vi "spectrum_display.vi"(4 "Chart data?":bool, 5 "Modulation info":T8 {"Hi channels at low" min=0 step=1; "Low carriers" format="%#_6p"; "High carriers" format="%#_6p"}, 6 "Reset STFT":bool, 7 "Config":T2={"IO params"={"Conversion"={"Rate"=0.0, "Num cards"=0, "Out channels"=4}, "Carriers"={"Phase shift"=180.0, "Levels"=[[0.8, 0.8, 0.8], [0.03, 0.03, 0.03]], "Delay samples"=73.15}, "TCP"={"Host"="192.168.1.15", "Port"=6666, "Buffering"=6, "Timeout"=6}, "Input channel sign"=[1, 1, 1]}, "High rate STFT"={"Win param"=0.0, "Window type"=0, "Win order"=0, "DFT size"=0, "Channels"=[], "Oversample"=0}, "Low rate STFT"={"Win param"=0.0, "Window type"=0, "Win order"=0, "DFT size"=0, "Channels"=[], "Oversample"=0}, "Filtering "=[]} {"Filtering"."Distortion"."Limit" format="%#_3p"; "Filtering"."Distortion"."LF cut" format="%#_3p"; "Filtering"."Kalman"."Measure noise" format="%#_3p"; "Filtering"."Kalman"."Process noise" format="%#_3p"; "Filtering"."Hum"."Limit" format="%#_3p"; "Filtering"."Hum"."Frequency" format="%#_4p"; "Low rate STFT"."Oversample" min=1 step=1; "Low rate STFT"."Channels" min=0 step=1; "Low rate STFT"."DFT size" min=1 step=1; "Low rate STFT"."Window type" items=["Rectangle"=0, "Hanning"=1, "Hamming"=2, "Blackman-Harris"=3, "Exact Blackman"=4, "Blackman"=5, "Flat Top"=6, "4 Term B-Harris "=7, "7 Term B-Harris"=8, "Low Sidelobe"=9, "Blackman Nuttall"=11, "Triangle"=30, "Bartlett-Hanning"=31, "Bohman"=32, "Parzen"=33, "Welch"=34, "Kaiser"=60, "Dolph-Chebyshev"=61, "Gaussian"=62]; "High rate STFT"."Oversample" min=1 step=1; "High rate STFT"."Channels" min=0 step=1; "High rate STFT"."DFT size" min=1 step=1; "High rate STFT"."Window type" items=["Rectangle"=0, "Hanning"=1, "Hamming"=2, "Blackman-Harris"=3, "Exact Blackman"=4, "Blackman"=5, "Flat Top"=6, "4 Term B-Harris "=7, "7 Term B-Harris"=8, "Low Sidelobe"=9, "Blackman Nuttall"=11, "Triangle"=30, "Bartlett-Hanning"=31, "Bohman"=32, "Parzen"=33, "Welch"=34, "Kaiser"=60, "Dolph-Chebyshev"=61, "Gaussian"=62]; "IO params"."Input channel sign" min=-1 max=1 step=1; "IO params"."Carriers"."Levels" min=0.0 step=0.1; "IO params"."Conversion"."Rate" format="%#_8g"}, 9 "Restart Averaging":bool, 10 "Spectrum parameters":T1={"Window"=enum."7 Term B-Harris", "FFT blocking"=enum."1", "Averaging"=5.0, "Order"=2} {"Order" min=1 max=100; "Averaging" min=0.0 max=1000.0 step=1.0}, 11 "Time domain wavevorms":waveform(dbl)[](array[waveform])) -> (2 "Complex spectrum":waveform(cdb)[](array[waveform]), 3 "dB spectrum":waveform(dbl)[](array[waveform]))   [LabVIEW 2026]
uses:
  processing/modulation_info.ctl
  processing/ilemt_config.ctl
  system/IO_params.ctl
  processing/stft_params.ctl
  <vilib>/Analysis/4window.llb/windowTd.ctl
  processing/filter_params.ctl
  processing/detrend_mode.ctl
  spectrum_parameters.ctl
  <vilib>/Analysis/NI_AALPro.lvlib
panel:
  out "time-freq sample info":cluster{"time steps":i32, "frequency bins":i32}
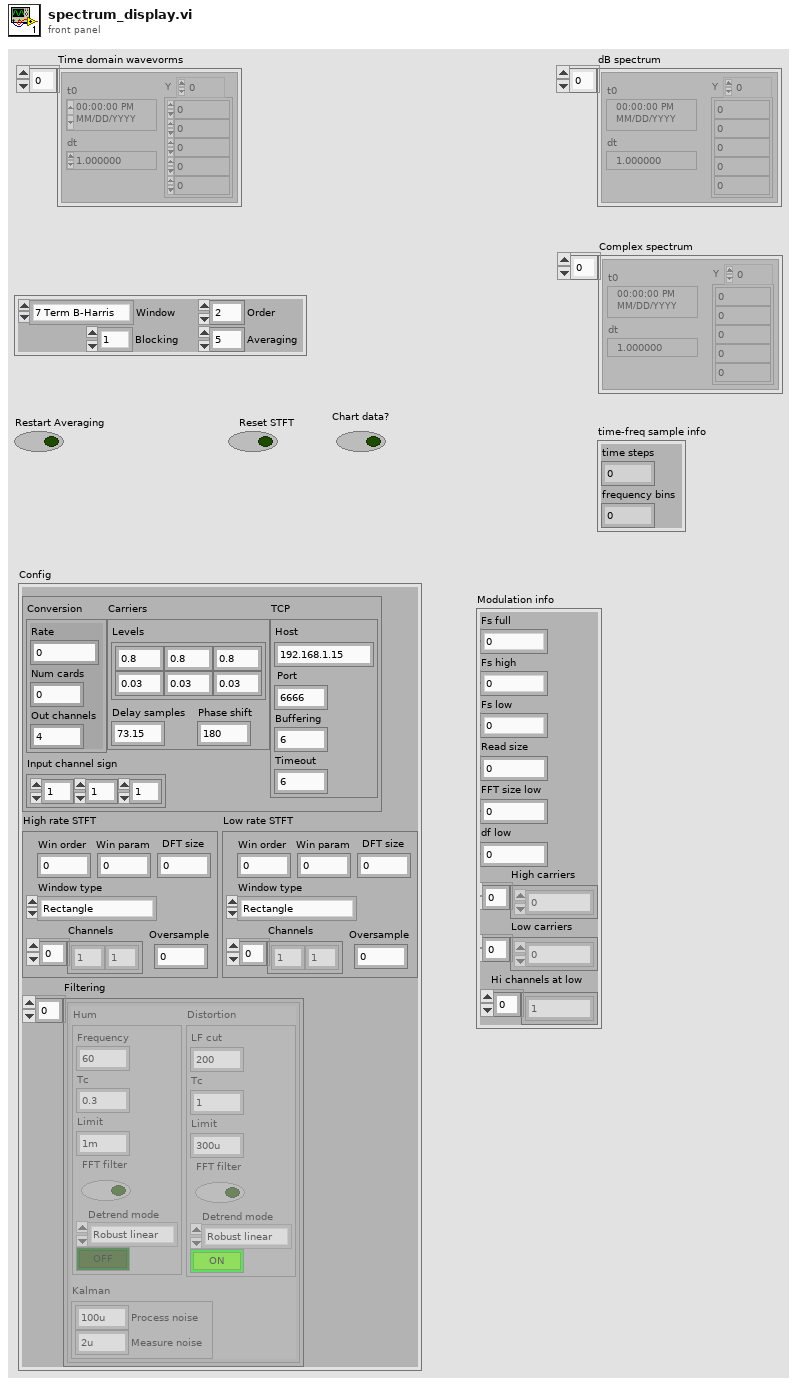
[diagram p1: front panel]
types:
  T1 = typedef "spectrum_parameters.ctl" = cluster{"Window":enum16{"None ", "Hanning", "Hamming", "Blackman-Harris", "Exact Blackman", "Blackman", "Flat Top", "4 Term B-Harris ", "7 Term B-Harris", "Low Sidelobe"}, "FFT blocking":enum16{"1", "2", "4", "8"}, "Averaging":dbl, "Order":u32}
  T2 = typedef "ilemt_config.ctl" = cluster{"IO params":T3, "High rate STFT":T4, "Low rate STFT":T4, "Filtering ":T6[]}
  T3 = typedef "IO_params.ctl" = cluster{"Conversion":cluster{"Rate":dbl, "Num cards":u32, "Out channels":u32}, "Carriers":cluster{"Phase shift":dbl, "Levels":dbl[][], "Delay samples":dbl}, "TCP":cluster{"Host":string, "Port":i32, "Buffering":u32, "Timeout":u32}, "Input channel sign":i32[]}
  T4 = typedef "stft_params.ctl" = cluster{"Win param":dbl, "Window type":T5, "Win order":i32, "DFT size":i32, "Channels":i32[], "Oversample":i32}
  T5 = typedef "NI_AALPro.lvlib/windowTd.ctl" = u32
  T6 = typedef "filter_params.ctl" = cluster{"Hum":cluster{"Frequency":dbl, "Tc":dbl, "Limit":dbl, "FFT filter":bool, "Detrend mode":T7, "Enable":bool}, "Kalman":cluster{"Process noise":dbl, "Measure noise":dbl}, "Distortion":cluster{"LF cut":dbl, "Tc":dbl, "Limit":dbl, "FFT filter":bool, "Detrend mode":T7, "Enable":bool}}
  T7 = typedef "detrend_mode.ctl" = enum16{"Zero mean", "Linear", "Robust linear"}
  T8 = typedef "modulation_info.ctl" = cluster{"Fs full":dbl, "Fs high":dbl, "Fs low":dbl, "Read size":i32, "FFT size low":i32, "df low":dbl, "High carriers":dbl[], "Low carriers":dbl[], "Hi channels at low":i32[]}
  T9 = enum16{"None ", "Hanning", "Hamming", "Blackman-Harris", "Exact Blackman", "Blackman", "Flat Top", "4 Term B-Harris ", "7 Term B-Harris", "Low Sidelobe"}
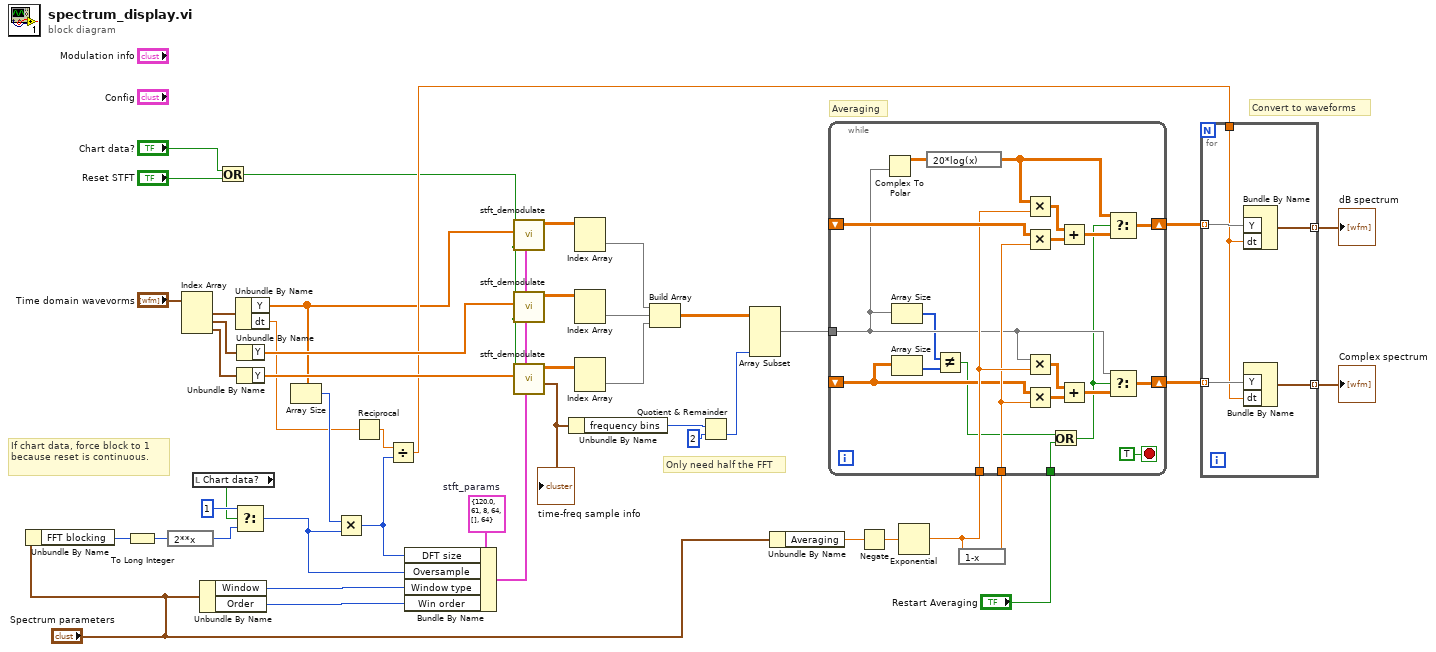
[diagram p0: block diagram]
diagram:
  w18 = T4 {"Win param"=120.0, "Window type"=61, "Win order"=8, "DFT size"=64, "Channels"=[], "Oversample"=64}  # stft_params
  # "If chart data, force block to 1 because reset is continuous."
  # "Convert to waveforms"
  # "Averaging"
  # "Only need half the FFT"
  n1 = Unbundle By Name("Spectrum parameters") -> ("FFT blocking"=w6:enum16{"1", "2", "4", "8"})
  n2 = To Long Integer(number=w6) -> (32bit integer=w5:i32)
  n3 = expression code="2**x"(w5) -> (w7:i32)
  n4 = Index Array(array="Time domain wavevorms") -> (element #1=w45:waveform(dbl), element #2=w44:waveform(dbl), element #3=w43:waveform(dbl))  [unwired: 3 in]
  n5 = local read "Chart data?"() -> (w3:bool)
  n6 = Unbundle By Name("Spectrum parameters") -> ("Window"=w40:T9, "Order"=w39:u32)
  n7 = Or(x="Chart data?", y="Reset STFT") -> (x .or. y?=w8:bool)
  n8 = Select(t=1, s=w3, f=w7) -> (s? t:f=w1:i32)
  n9 = Unbundle By Name(w45) -> ("Y"=w12:dbl[], "dt"=w11:dbl)
  n10 = Unbundle By Name(w44) -> ("Y"=w42:dbl[])
  n11 = Unbundle By Name(w43) -> ("Y"=w15:dbl[])
  n12 = Array Size(array=w12) -> (size(s)=w17:i32)
  n13 = Multiply(x=w17, y=w1) -> (x*y=w14:i32)
  n14 = Reciprocal(x=w11) -> (1/x=w41:dbl)
  n15 = Divide(x=w41, y=w14) -> (x/y=w13:dbl)
  n16 = Bundle By Name(cluster=w18, "DFT size"=w14, "Oversample"=w1, "Window type"=w40, "Win order"=w39) -> (w46:T4)
  n17 = call "stft_demodulate.vi"("STFT params"=w46, "Reset"=w8, "X"=w12) -> ("STFT"=w38:cdb[][])  [unwired: 6 in, 2 out]
  n18 = call "stft_demodulate.vi"("STFT params"=w46, "Reset"=w8, "X"=w42) -> ("STFT"=w37:cdb[][])  [unwired: 6 in, 2 out]
  n19 = call "stft_demodulate.vi"("STFT params"=w46, "Reset"=w8, "X"=w15) -> ("time-freq sample info"=w26:cluster{"time steps":i32, "frequency bins":i32}, "STFT"=w36:cdb[][])  [unwired: 6 in, 1 out]
  "time-freq sample info" <- w26
  n20 = Unbundle By Name(w26) -> ("frequency bins"=w25:i32)
  n21 = Index Array(array=w38) -> (element=w35:cdb[])  [unwired: 2 in]
  n22 = Index Array(array=w37) -> (element=w34:cdb[])  [unwired: 2 in]
  n23 = Index Array(array=w36) -> (element=w33:cdb[])  [unwired: 2 in]
  n24 = Build Array(w35, w34, w33) -> (w27:cdb[][])
  n25 = Quotient & Remainder(x=w25, y=2) -> (floor(x/y)=w24:i32)  [unwired: 1 out]
  n26 = Array Subset(array=w27, length (col)=w24) -> (w23:cdb[][])  [unwired: 3 in]
  n27 = Unbundle By Name("Spectrum parameters") -> ("Averaging"=w32:dbl)
  n28 = Negate(x=w32) -> (-x=w31:dbl)
  n29 = Exponential(1:w31) -> (0:w30:dbl)
  n30 = expression code="1-x"(w30) -> (w29:dbl)
  n31 = while {
    tunnel: w30 -> [w56]
    tunnel: w29 -> [w55]
    shift-right: [w67] -> w22
    shift-left: _ -> [w61]
    tunnel: "Restart Averaging" -> [w49]
    tunnel: w23 -> [w54]
    shift-right: [w57] -> w21
    shift-left: _ -> [w53]
    stop <- TRUE stop-if-true
    n32 = Complex To Polar(r * e^(i*theta)=w54) -> (r=w68:dbl[][])  [unwired: 1 out]
    n33 = Array Size(array=w54) -> (size(s)=w51:i32[])
    n34 = Array Size(array=w53) -> (size(s)=w52:i32[])
    n35 = expression code="20*log(x)"(w68) -> (w64:dbl[][])
    n36 = Not Equal?(x=w51, y=w52) -> (x != y?=w50:bool)
    n37 = Multiply(x=w64, y=w56) -> (x*y=w66:dbl[][])
    n38 = Multiply(x=w61, y=w55) -> (x*y=w65:dbl[][])
    n39 = Multiply(x=w54, y=w56) -> (x*y=w58:cdb[][])
    n40 = Multiply(x=w53, y=w55) -> (x*y=w59:cdb[][])
    n41 = Or(x=w50, y=w49) -> (x .or. y?=w48:bool)
    n42 = Add(x=w66, y=w65) -> (x+y=w63:dbl[][])
    n43 = Add(x=w58, y=w59) -> (x+y=w60:cdb[][])
    n44 = Select(t=w64, s=w48, f=w63) -> (s? t:f=w67:dbl[][])
    n45 = Select(t=w54, s=w48, f=w60) -> (s? t:f=w57:cdb[][])
  }
  n46 = for {
    tunnel: w22 -> [w73] mode=indexing
    tunnel: w21 -> [w71] mode=indexing
    tunnel: w13 -> [w69]
    tunnel: [w72] -> w20 mode=indexing
    tunnel: [w70] -> w19 mode=indexing
    n47 = Bundle By Name("Y"=w73, "dt"=w69) -> (w72:waveform(dbl))  [unwired: 1 in]
    n48 = Bundle By Name("Y"=w71, "dt"=w69) -> (w70:waveform(cdb))  [unwired: 1 in]
  }
  "Complex spectrum" <- w19
  "dB spectrum" <- w20
